vi "RSZVB Get Sweep Segment Meas Bandwidth.vi"(8 "error in (no error)":errorcluster {"code" format="%.0x"}, 9 "Segment (1)":i32=1, 10 "Channel (1)":i32=1, 11 "VISA session":refnum<visa-resource-name>) -> (0 "error out":errorcluster {"code" format="%.0x"}, 2 "Meas Bandwidth":dbl format="%^.3e", 3 "dup VISA session":refnum<visa-resource-name>)   [LabVIEW 2011]
doc: "This VI queries the resolution bandwidth of the analyzer in sweep segment no. <Segment>. At the same time, the command activates separate bandwidth setting in all sweep segments.\n\nRemote-control command(s):\n[SENSe<Ch>:]SEGMent<Seg>:BWIDth[:RESolution]?"
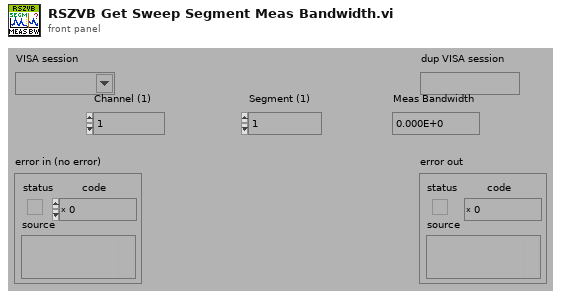
[diagram p1: front panel]
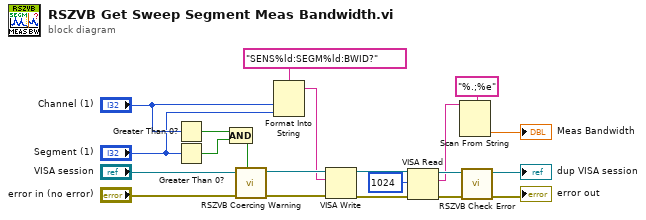
[diagram p0: block diagram]
diagram:
  n1 = Greater Than 0?(x="Channel (1)") -> (x > 0?=w12:bool)
  n2 = Greater Than 0?(x="Segment (1)") -> (x > 0?=w11:bool)
  n3 = Compound Arithmetic op=AND(w12, w11) -> (w14:bool)
  n4 = call "RSZVB Coercing Warning.vi"("In Range?"=w14, "error in (no error)"="error in (no error)", "VISA session"="VISA session") -> ("error out"=w15:errorcluster, "dup VISA session"=w16:refnum<visa-resource-name>)  [unwired: 7 in]
  n5 = Format Into String(format string="SENS%ld:SEGM%ld:BWID?", "Channel (1)", "Segment (1)") -> (resulting string=w13:string)  [unwired: 2 in, 1 out]
  n6 = VISA Write(VISA resource name=w16, write buffer=w13, error in (no error)=w15) -> (VISA resource name out=w9:refnum<visa-resource-name>, error out=w10:errorcluster)  [unwired: 1 out]
  n7 = VISA Read(VISA resource name=w9, byte count=u32 1024 ("byte count (0)"), error in (no error)=w10) -> (VISA resource name out=w21:refnum<visa-resource-name>, read buffer=w18:string, error out=w20:errorcluster)  [unwired: 1 out]
  n8 = Scan From String(format string="%.;%e", input string=w18) -> (output 1=→"Meas Bandwidth":dbl)  [unwired: 3 in, 3 out]
  n9 = call "RSZVB Check Error.vi"("error in (no error)"=w20, "VISA session"=w21) -> ("error out"=→"error out":errorcluster, "dup VISA session"=→"dup VISA session":refnum<visa-resource-name>)  [unwired: 8 in]
